vi "Configure Division.vi"(8 "error in (no error)":errorcluster, 9 "Division factor (5)":dbl=5.0 format="%#_9g", 10 "Enable Division (T: ON)":bool=TRUE, 11 "VISA resource name":refnum<visa-resource-name>) -> (0 "error out":errorcluster, 3 "VISA resource name out":refnum<visa-resource-name>)   [LabVIEW 2011, in "Fluke 8508.lvlib"]
doc: "This VI sets the division function on the instrument and configures the division factor.\n\nCombinations of math VIs are allowed, but they must be performed in the following order:\n1. Averaging\n2. Multiplication \n3. Subtraction \n4. Division\n5. Decibels"
uses:
  Fluke 8508.lvlib
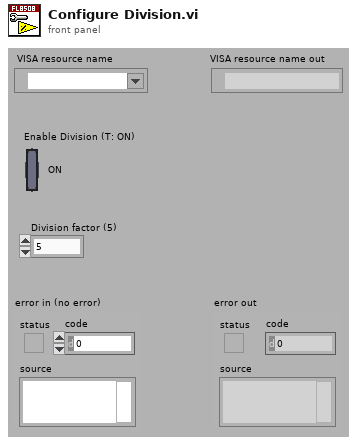
[diagram p1: front panel]
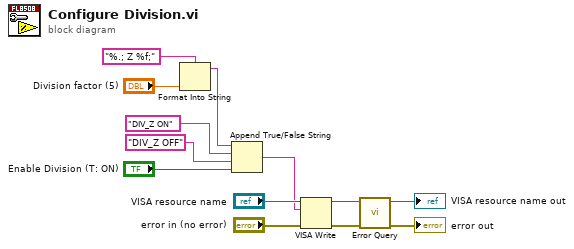
[diagram p0: block diagram]
diagram:
  n1 = Format Into String(format string="%.; Z %f;", "Division factor (5)") -> (resulting string=w8:string)  [unwired: 2 in, 1 out]
  n2 = Append True/False String(1:"Enable Division (T: ON)", 2:"DIV_Z OFF" ("true string"), 3:"DIV_Z ON" ("true string"), 4:w8) -> (0:w5:string)
  n3 = VISA Write(VISA resource name="VISA resource name", write buffer=w5, error in (no error)="error in (no error)") -> (VISA resource name out=w3:refnum<visa-resource-name>, error out=w4:errorcluster)  [unwired: 1 out]
  n4 = call "Error Query.vi"("error in (no error)"=w4, "VISA resource name"=w3) -> ("error out"=→"error out":errorcluster, "VISA resource name out"=→"VISA resource name out":refnum<visa-resource-name>)  [unwired: 6 in, 2 out]
